vi "Read.vi"(7 "timeout (100ms)":i32=100, 8 "error in (no error)":errorcluster, 9 "Interlock in":bool, 11 "Interlock Sample in":refnum<class "Interlock Sample.lvclass">) -> (0 "error out":errorcluster, 1 "Interlock out":bool, 2 "Data out":variant, 3 "Interlock Sample out":refnum<class "Interlock Sample.lvclass">, 4 "IL Action":refnum<class "IL Action.lvclass">[](array[class]))   [LabVIEW 2015, in "Interlocks.lvlib" / "Interlock Sample.lvclass"]
uses:
  Interlock Sample.lvclass
  IL Action/IL Action.lvclass
  Interlock Sample.lvclass/Interlock Sample.ctl
  Interlock/State Enum.ctl
  Interlock/Interlock.lvclass/Interlock.ctl
  subs/Sample/Sample.lvclass
  Interlock/Interlock.lvclass
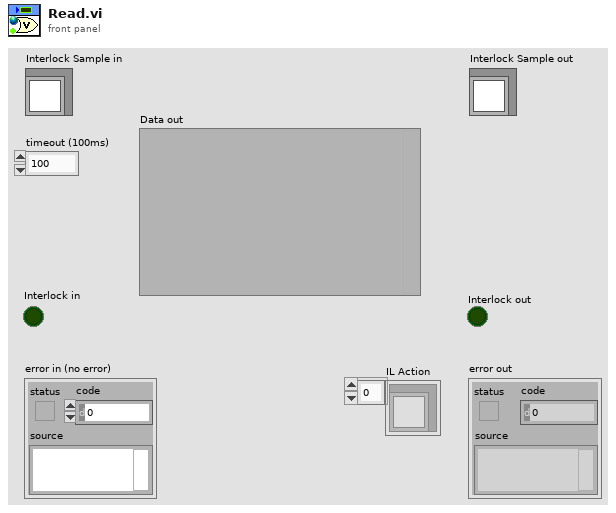
[diagram p1: front panel]
types:
  T1 = typedef "Interlocks.lvlib/Interlock.lvclass/State Enum.ctl" = enum16{"Error", "Ok", "Interlock", "Out of Range", "Is ON", "Is OFF", "Denied", "Not Allowed", "Sample Allow", "Sample Deny"}
  T2 = typedef "Action Enum.ctl" = enum16{"Allow", "Deny"}
  T3 = typedef "Sample Container.ctl" = cluster{"Sample In":refnum<k21>, "Sample Name":refnum<k21>, "Ti Cathode":refnum<k21>, "SampleQ":refnum<queue>}
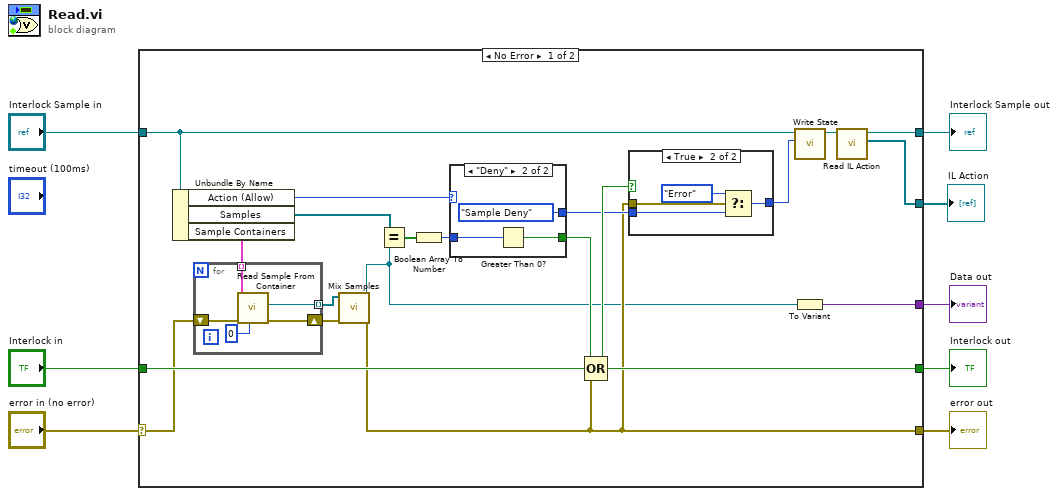
[diagram p0: block diagram]
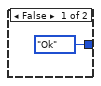
[diagram p2: hidden frame]
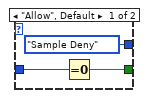
[diagram p3: hidden frame]
diagram:
  n1 = case shown="No Error" "error in (no error)" {
    selector: "error in (no error)" -> [w16 w45]
    tunnel: "Interlock Sample in" -> [w20 w46]
    tunnel: [w14 w45] -> w7
    tunnel: "Interlock in" -> [w23 w47]
    tunnel: [w21 w47] -> w4
    tunnel: [w10 w46] -> w3
    tunnel: [w18 _] -> w2
    tunnel: [w9 _] -> w1
    frame No Error {
      n2 = Unbundle By Name(w20) -> ("Action (Allow)"=w24:T2, "Samples"=w27:refnum<class "Sample.lvclass">[], "Sample Containers"=w28:T3[])
      n3 = for {
        tunnel: w28 -> [w33] mode=indexing
        tunnel: [w30] -> w13 mode=indexing
        shift-right: [w31] -> w15
        shift-left: w16 -> [w32]
        n4 = call "Read Sample From Container.vi"("Queue timeout in ms (-1)"=0, "error in (no error)"=w32, "Container"=w33) -> ("error out"=w31:errorcluster, "Sample out"=w30:refnum<class "Sample.lvclass">)  [unwired: 4 in, 3 out]
      }
      n5 = call "Mix Samples.vi"("error in (no error)"=w15, "Samples In"=w13) -> ("error out"=w14:errorcluster, "Sample out"=w12:refnum<class "Sample.lvclass">)  [unwired: 6 in, 2 out]
      n6 = Equal?(x=w27, y=w12) -> (x = y?=w26:bool[])
      n7 = Boolean Array To Number(Boolean array=w26) -> (number=w25:u32)
      n8 = case shown="\"Deny\"" w24 {
        tunnel: [w41 w43] -> w22
        tunnel: w25 -> [w40 w44]
        tunnel: [State_Enum."Sample Deny" ("State") State_Enum."Sample Deny" ("State")] -> w17
        frame "Allow", Default {
          n9 = Equal To 0?(x=w40) -> (x = 0?=w41:bool)
        }
        frame "Deny" {
          n10 = Greater Than 0?(x=w44) -> (x > 0?=w43:bool)
        }
      }
      n11 = Compound Arithmetic op=OR(w22, w23, w14) -> (w21:bool)
      n12 = case shown="True" w21 {
        tunnel: w14 -> [_ w38]
        tunnel: [State_Enum."Ok" ("State") w36] -> w19
        tunnel: w17 -> [_ w35]
        frame False {
        }
        frame True {
          n13 = Select(t=State_Enum."Error", s=w38, f=w35) -> (s? t:f=w36:T1)
        }
      }
      n14 = call "Write State.vi"("State"=w19, "Interlock in"=w20) -> ("Interlock out"=w11:refnum<class "Interlock Sample.lvclass">)  [unwired: 9 in]
      n15 = To Variant(anything=w12) -> (Variant=w18:variant)
      n16 = call "Read IL Action.vi"("Interlock in"=w11) -> ("IL Action"=w9:refnum<class "IL Action.lvclass">[], "Interlock out"=w10:refnum<class "Interlock Sample.lvclass">)  [unwired: 9 in]
    }
    frame Error {
    }
  }
  "error out" <- w7
  "Interlock Sample out" <- w3
  "Data out" <- w2
  "Interlock out" <- w4
  "IL Action" <- w1
